vi "Read T Controller Settings.vi"(8 "error in (no error)":errorcluster, 11 "LakeShore 340 in":refnum<class "LakeShore 340.lvclass">) -> (0 "error out":errorcluster, 1 "Heater level":dbl, 2 "Heater mode":T1(ring), 3 "LakeShore 340 out":refnum<class "LakeShore 340.lvclass">, 4 "PID":cluster{"P":dbl, "I":dbl, "D":dbl}, 5 "Hater range":dbl, 7 "Set point":dbl)   [LabVIEW 2015, in "LakeShore 340.lvclass"]
uses:
  LakeShore 340.lvclass
  Instrument/Instrument.lvclass
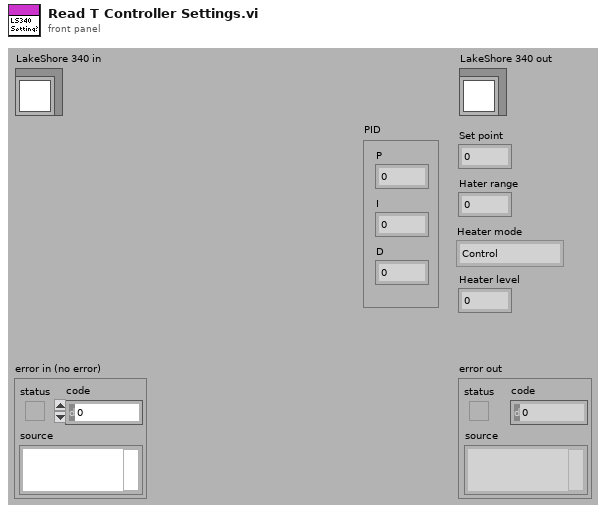
[diagram p1: front panel]
types:
  T1 = enum16{"Control", "Monitor", "Manual Heat", "Controller is in OFF mode", "Autotune is in progress"}
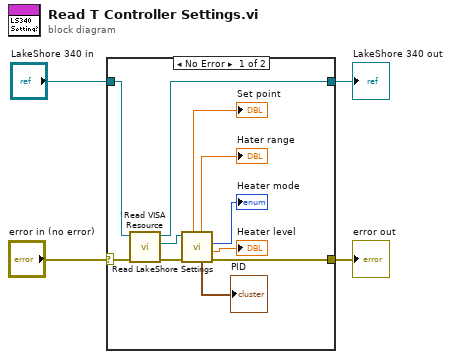
[diagram p0: block diagram]
diagram:
  n1 = case shown="No Error" "error in (no error)" {
    selector: "error in (no error)" -> [w13 w17]
    tunnel: [w6 w17] -> w3
    tunnel: [w14 w16] -> w1
    tunnel: "LakeShore 340 in" -> [w15 w16]
    frame No Error {
      n2 = call "Read VISA Resource.vi"("error in (no error)"=w13, "Instrument.lvclass in"=w15) -> ("error out"=w7:errorcluster, "VISA Resource"=w8:refnum<visa-resource-name>, "Instrument.lvclass out"=w14:refnum<class "LakeShore 340.lvclass">)  [unwired: 7 out]
      n3 = call "Read LakeShore Settings.vi"("error in (no error)"=w7, "VISA resource name"=w8) -> ("error out"=w6:errorcluster, "Heater level"=→"Heater level":dbl, "Heater mode"=→"Heater mode":T1, "PID"=→"PID":cluster{"P":dbl, "I":dbl, "D":dbl}, "Hater range"=→"Hater range":dbl, "Set point"=→"Set point":dbl)  [unwired: 3 in, 1 out]
    }
    frame Error {
    }
  }
  "error out" <- w3
  "LakeShore 340 out" <- w1
